vi "Get Frequency.vi"(8 "error in (no error)":errorcluster, 11 "RP Instrument in":refnum<class "RP Instrument.lvclass">) -> (0 "error out":errorcluster, 2 "Frequency":u32=1 format="0x%x (%d)", 3 "RP Instrument out":refnum<class "RP Instrument.lvclass">)   [LabVIEW 2019, in "RP Instrument.lvclass"]
uses:
  RP Instrument.lvclass
  RP Config Offsets.ctl
  RP Instrument.lvclass/RP Instrument.ctl
  RP Communicator/RP Communicator.lvclass
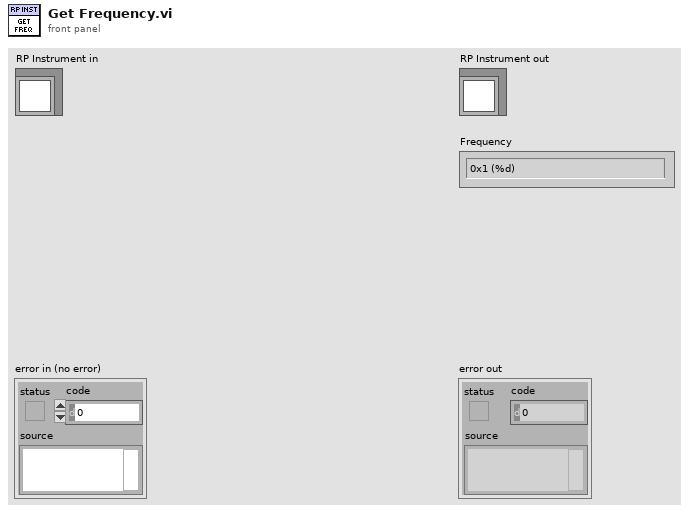
[diagram p1: front panel]
types:
  T1 = typedef "RP Config Offsets.ctl" = u16
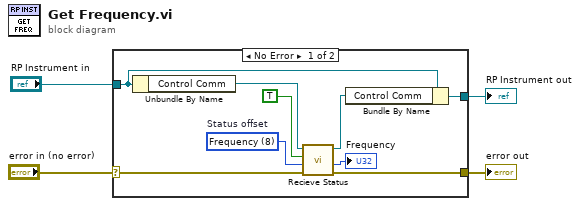
[diagram p0: block diagram]
diagram:
  n1 = case shown="No Error" "error in (no error)" {
    selector: "error in (no error)" -> [w9 w15]
    tunnel: [w8 w15] -> w3
    tunnel: [w5 w14] -> w1
    tunnel: "RP Instrument in" -> [w6 w14]
    frame No Error {
      w10 = T1 8 items=["Config flags"=0, "Record length"=4, "Frequency"=8, "Decimation"=12, "LED"=16, "DDS delay"=28]  # Status offset
      n2 = Unbundle By Name(w6) -> ("Control Comm"=w13:refnum<class "RP Communicator.lvclass">)
      n3 = call-dynamic "Recieve Status.vi"("error in (no error)"=w9, "Status offset"=w10, "Read config instead"=TRUE, "RP Communicator in"=w13) -> ("error out"=w8:errorcluster, "Status response"=→"Frequency":u32, "RP Communicator out"=w12:refnum<class "RP Communicator.lvclass">)  [unwired: 5 in]
      n4 = Bundle By Name(cluster=w6, "Control Comm"=w12) -> (w5:refnum<class "RP Instrument.lvclass">)
    }
    frame Error {
    }
  }
  "error out" <- w3
  "RP Instrument out" <- w1
